vi "3.2.vi"() -> ()   [LabVIEW 2018]
panel:
  out "이후 부분 문자열":string
  out "길이":dbl
  out "결과문":string
  in  "맺음말":string
  in  "머리말":string
  out "결과":string
  out "결과":dbl
  in  "난이도":dbl
  in  "독창성":dbl
  in  "창의력":dbl
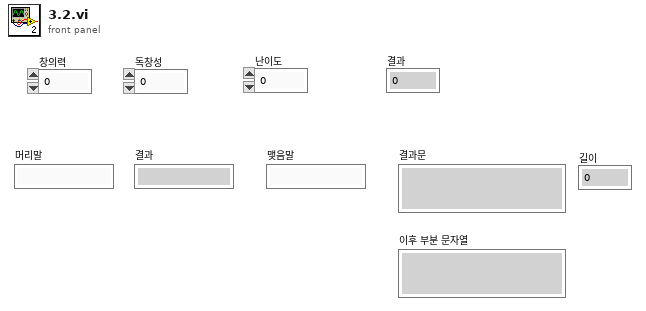
[diagram p1: front panel]
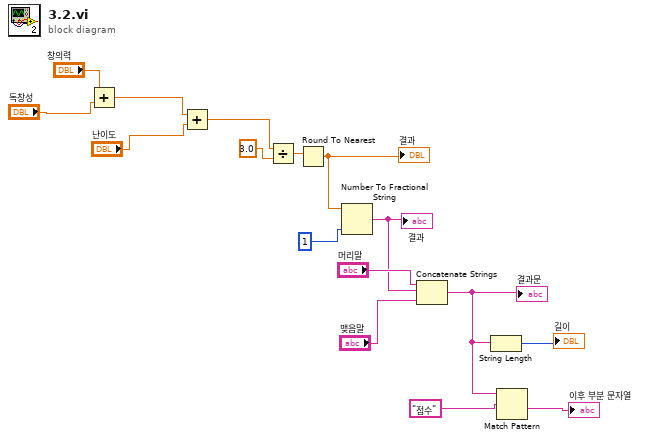
[diagram p0: block diagram]
diagram:
  n1 = Add(x="창의력", y="독창성") -> (x+y=w14:dbl)
  n2 = Add(x=w14, y="난이도") -> (x+y=w12:dbl)
  n3 = Divide(x=w12, y=3.0 ("x")) -> (x/y=w11:dbl)
  n4 = Round To Nearest(number=w11) -> (nearest integer value=w9:dbl)
  "결과" <- w9
  n5 = Number To Fractional String(number=w9, precision (6)=1) -> (F-format string=w6:string)  [unwired: 2 in]
  "결과" <- w6
  n6 = Concatenate Strings("머리말", w6, "맺음말") -> (w3:string)
  "결과문" <- w3
  n7 = String Length(string=w3) -> (length=→"길이":i32)
  n8 = Match Pattern(string=w3, regular expression="점수") -> (after substring=→"이후 부분 문자열":string)  [unwired: 1 in, 3 out]
